vi "Grab (177x Smart Camera).vi"() -> ()   [LabVIEW 2011]
doc: "The Grab (177x Smart Camera) VI performs a high-level grab acquisition and exposes control of the sensor interface for NI 177x Series devices. A grab is appropriate for high-speed applications that process only one image at a time.\n\nUse the Sensor Parameters cluster to control attributes related to the sensor. Use the Exposure Time control (in microseconds) to precisely control the amount of time that the image sensor is sensitive to light. Use the Gain control to determine the gain of the camera. Use the Reverse X and Reverse Y to flip the image horizontally or vertically.\n\nUse the Lighting Parameters cluster to control the internal lighting controller. The internal lighting controller is precisely synchronized with the exposure of the image sensor. This guarantees that the light is on for the duration of the image exposure period.\n\nUse the Trigger Parameters cluster to configure the trigger mode of the acquisition. These settings must be configured before running the VI because they are ignored while the acquisition is active."
uses:
  <vilib>/vision/driver/IMAQdx.llb/IMAQdx Buffer Number Mode.ctl
  <vilib>/vision/driver/NI_Vision_Acquisition_Software.lvlib
  <vilib>/vision/driver/IMAQdx.llb/IMAQdx Acquisition Mode.ctl
  resource/objmgr/imaqdx.rc
panel:
  in  "SW Trigger":bool
  in  "Trigger Parameters":T1={"Trigger Mode"="Off", "Trigger Source"="External Trigger", "Fixed Frame Rate"=0.25, "Timeout (ms)"=5000, "Trigger Delay (us)"=0.0} {"Trigger Delay (us)" min=0.0 max=4295000.0; "Fixed Frame Rate" min=0.25 max=15.0}
  in  "Lighting Parameters":cluster{"Mode":string, "Current Level (mA)":dbl}={"Mode"="Off", "Current Level (mA)"=0.0} {"Current Level (mA)" min=0.0 max=0.0 step=1.0 scale=0.0..100.0}
  in  "Color Parameters":T2 {"Gamma" scale=0.0..1.0; "Blue Gain" scale=0.0..3.99; "Green Gain" scale=0.0..3.99; "Red Gain" scale=0.0..3.99}
  in  "Sensor Parameters":T3={"Exposure Time (ms)"=50.0, "Gain"=0.0, "Reverse X"=FALSE, "Reverse Y"=FALSE} {"Gain" min=0.0 max=255.0; "Exposure Time (ms)" min=0.057798999999999996 max=2101.471043 scale=0.057798999999999996..1000.0 scale format="%#_1f"}
  in  "Camera Name":refnum<k21> caption="IMAQdx Session"
  out "Image":T4(plugin-control)
  out "Frame Rate":dbl(knob) scale=0.0..100.0
  in  "Stop":bool
  # "Overview: Demonstrates how to perform a high-level grab acquisition and control of the sensor interface for NI 177x Series devices.  \nRequirements: Vision Acquisition Software, NI 177x series smart camera. For 17xx cameras, use the examples in the NI-IMAQ folder instead.\nInstructions: \n1. Open a New LabVIEW Project. Select to Add this VI to the project when prompted.\n2. Right click on the Project in the tree and select New>>Targets and Devices...\n3. Select the Smart Camera you want to run this example with, and click OK.\n4. Drag this VI from My Computer to the Smart Camera.\n5. Double click on the example under the Smart Camera, select the Camera Name, and run the VI."
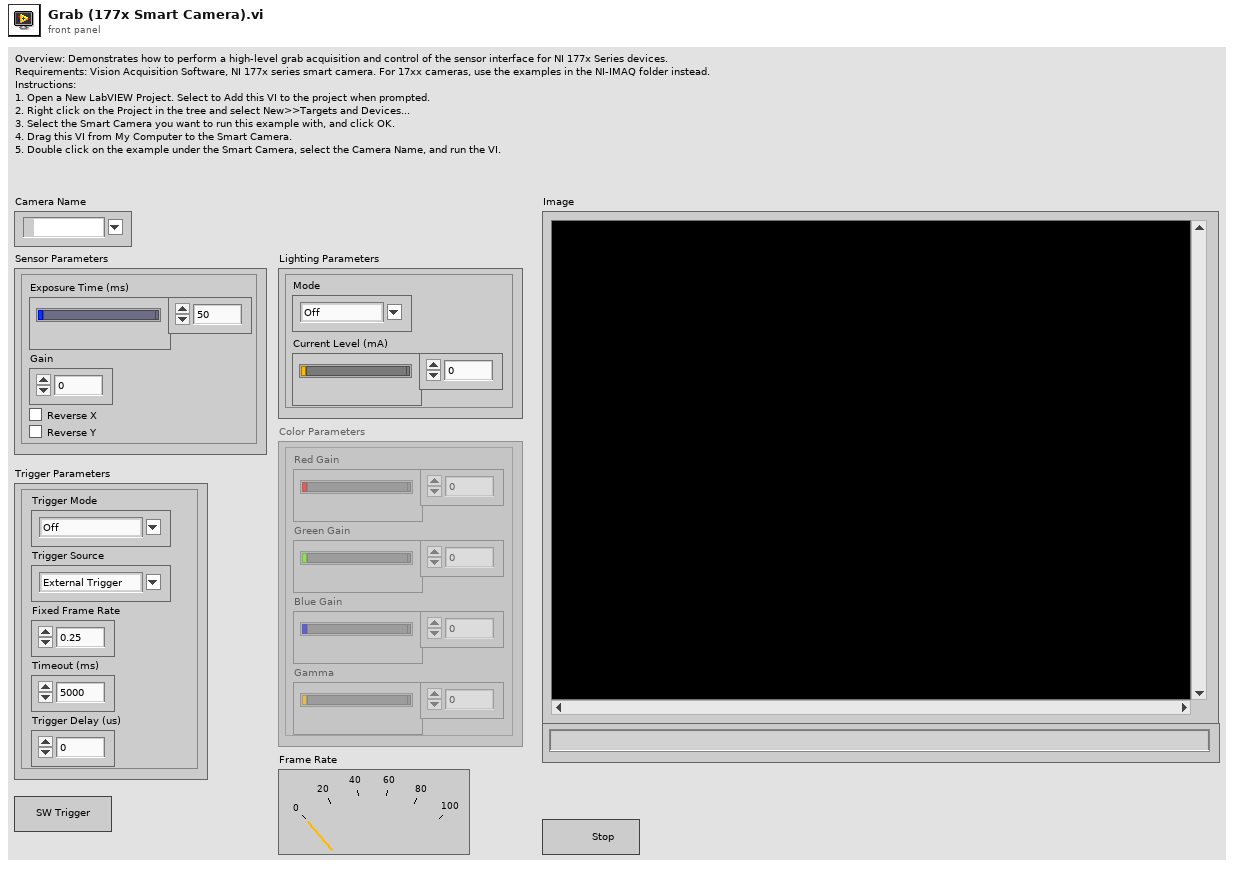
[diagram p1: front panel]
types:
  T1 = cluster{"Trigger Mode":string, "Trigger Source":string, "Fixed Frame Rate":dbl, "Timeout (ms)":u32, "Trigger Delay (us)":dbl}
  T2 = cluster{"Red Gain":dbl, "Green Gain":dbl, "Blue Gain":dbl, "Gamma":dbl}
  T3 = cluster{"Exposure Time (ms)":dbl, "Gain":dbl, "Reverse X":bool, "Reverse Y":bool}
  T4 = typedef "IMAQ Image.ctl" = refnum<image>
  T5 = enum8{"Enabled", "Disabled", "Disabled and Grayed Out"}
  T6 = typedef "NI_Vision_Acquisition_Software.lvlib/IMAQdx Acquisition Mode.ctl" = enum32{"One Shot", "Continuous"}
  T7 = typedef "IMAQdx.ctl" = refnum<k21>
  T8 = typedef "NI_Vision_Acquisition_Software.lvlib/IMAQdx Buffer Number Mode.ctl" = enum32{"Next", "Last", "Buffer Number", "Every", "Last New"}
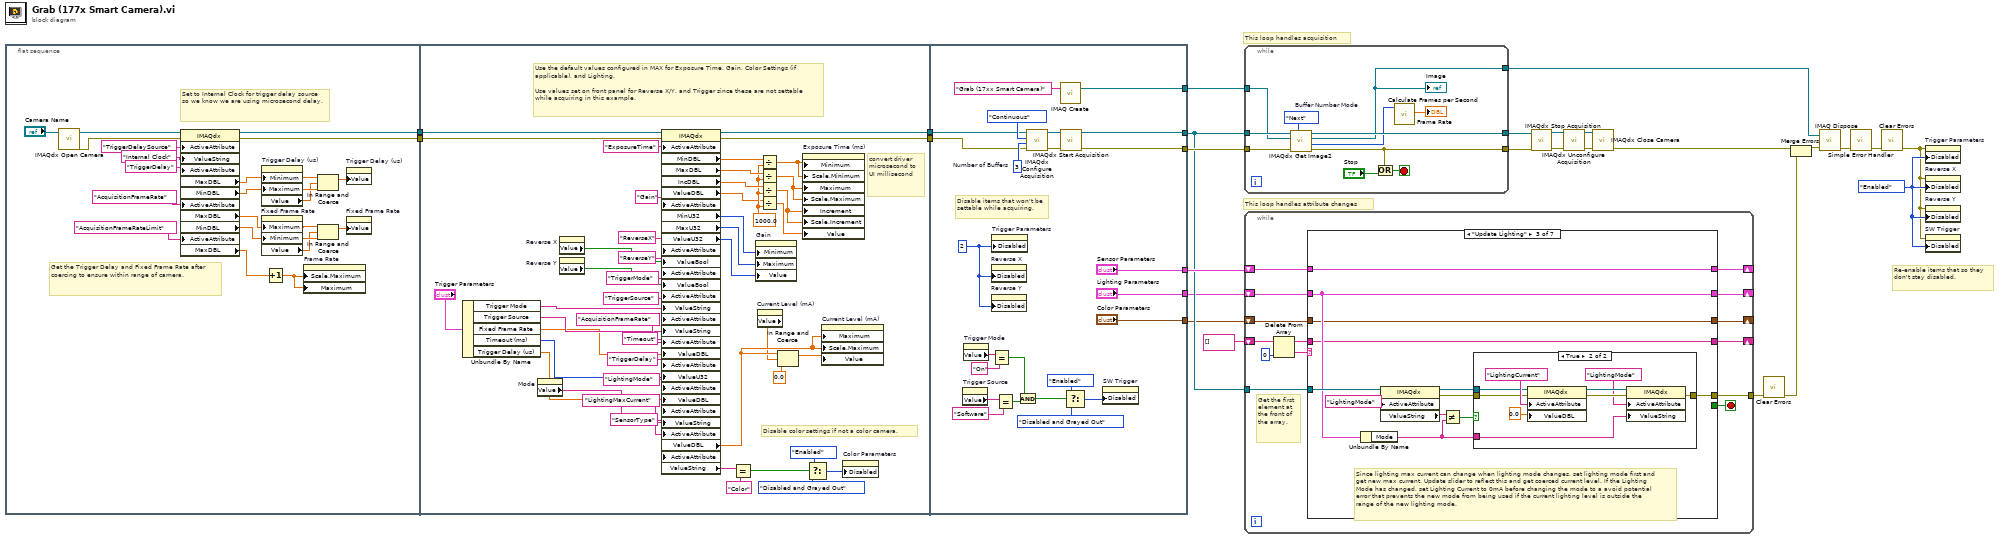
[diagram p0: block diagram]
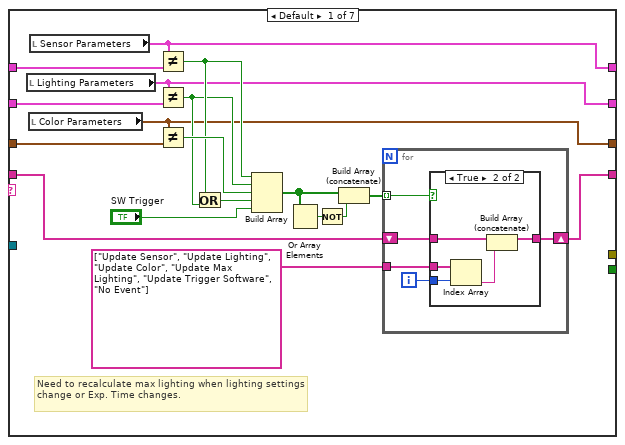
[diagram p2: hidden frame]
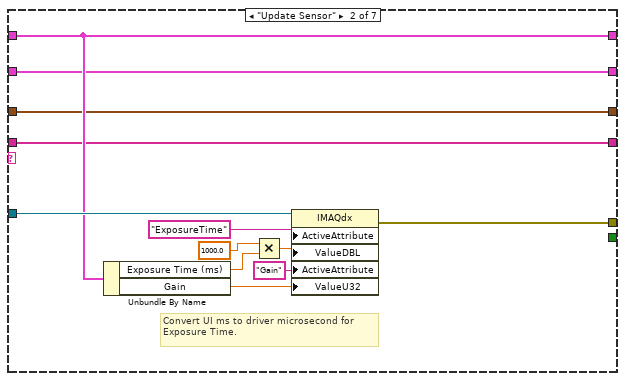
[diagram p4: hidden frame]
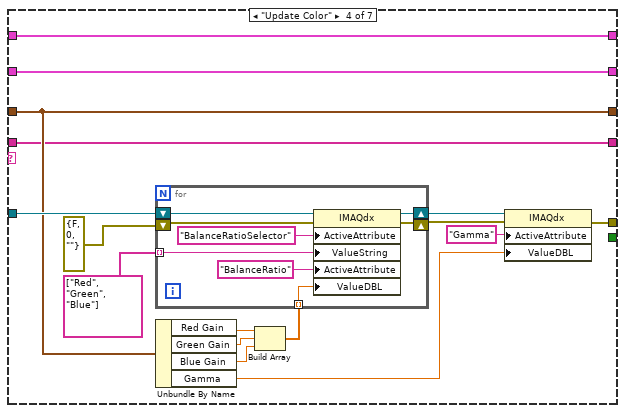
[diagram p6: hidden frame]
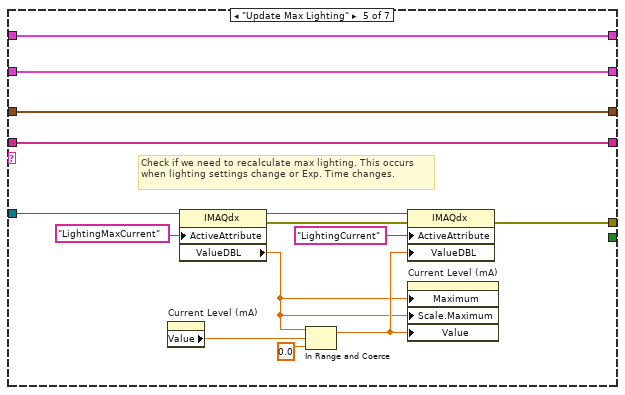
[diagram p7: hidden frame]
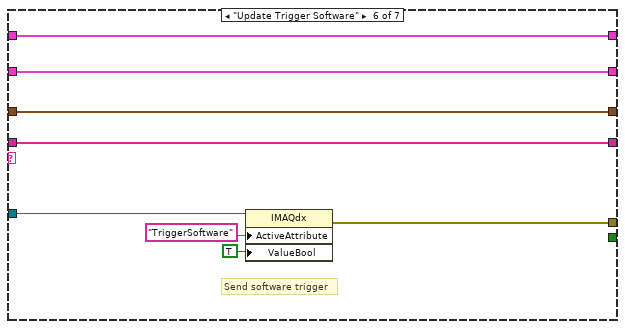
[diagram p8: hidden frame]
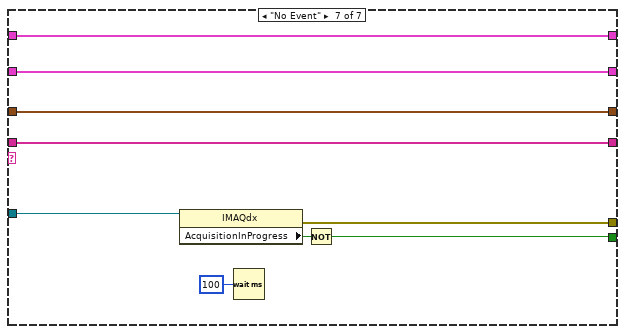
[diagram p9: hidden frame]
diagram:
  w12 = T5."Enabled" ("Disabled")
  # "Re-enable items that so they don't stay disabled."
  # "This loop handles acquisition"
  # "This loop handles attribute changes"
  n1 = flat-sequence {
    tunnel: [w30] -> w21
    tunnel: [w35] -> w20
    tunnel: w21 -> [w56]
    tunnel: [w55] -> w19
    tunnel: w20 -> [w83]
    tunnel: [w69] -> w18
    tunnel: w19 -> [w113]
    tunnel: [w111] -> w24
    tunnel: [w110] -> w26
    tunnel: ["Sensor Parameters"] -> w25
    tunnel: ["Lighting Parameters"] -> w23
    tunnel: ["Color Parameters"] -> w22
    tunnel: w18 -> [w112]
    tunnel: [w94] -> w17
    frame #0 {
      # "Get the Trigger Delay and Fixed Frame Rate after coercing to ensure within range of camera."
      # "Set to Internal Clock for trigger delay source so we know we are using microsecond delay."
      n2 = call <vilib>:"IMAQdx Open Camera.vi"("Session In"="Camera Name") -> ("error out"=w27:errorcluster, "Session Out"=w28:T7)  [unwired: 2 in, 7 out]
      n3 = property class="IMAQdx"(reference=w28, error in=w27, "ActiveAttribute"="TriggerDelaySource", "ValueString"="Internal Clock", "ActiveAttribute"="TriggerDelay", "ActiveAttribute"="AcquisitionFrameRate", "ActiveAttribute"="AcquisitionFrameRateLimit") -> (reference out=w30:T7, error out=w35:errorcluster, "MaxDBL"=w43:dbl, "MinDBL"=w42:dbl, "MaxDBL"=w38:dbl, "MinDBL"=w37:dbl, "MaxDBL"=w31:dbl)
      n4 = property on="Trigger Delay (us)" class="DigNum (strict)"("Minimum"=w43, "Maximum"=w42) -> ("Value"=w41:dbl)  [unwired: 2 in, 2 out]
      n5 = property on="Fixed Frame Rate" class="DigNum (strict)"("Maximum"=w38, "Minimum"=w37) -> ("Value"=w36:dbl)  [unwired: 2 in, 2 out]
      n6 = Increment(x=w31) -> (x+1=w32:dbl)
      n7 = property on="Frame Rate" class="Knob (strict)"("Scale.Maximum"=w32, "Maximum"=w32) -> ()  [unwired: 2 in, 2 out]
      n8 = In Range and Coerce(upper limit=w43, x=w41, lower limit=w42) -> (coerced(x)=w40:dbl)  [unwired: 1 out]
      n9 = In Range and Coerce(upper limit=w38, x=w36, lower limit=w37) -> (coerced(x)=w34:dbl)  [unwired: 1 out]
      n10 = property on="Trigger Delay (us)" class="DigNum (strict)"("Value"=w40) -> ()  [unwired: 2 in, 2 out]
      n11 = property on="Fixed Frame Rate" class="DigNum (strict)"("Value"=w34) -> ()  [unwired: 2 in, 2 out]
    }
    frame #1 {
      w63 = 1000.0 ("y")
      # "convert driver microsecond to UI millisecond"
      # "Disable color settings if not a color camera."
      # "Use the default values configured in MAX for Exposure Time, Gain, Color Settings (if applicable), and Lighting.\n\nUse values set on front panel for Reverse X/Y, and Trigger since these are not settable while acquiring in this example."
      n12 = Unbundle By Name("Trigger Parameters") -> ("Trigger Mode"=w47:string, "Trigger Source"=w51:string, "Fixed Frame Rate"=w50:dbl, "Timeout (ms)"=w49:u32, "Trigger Delay (us)"=w48:dbl)
      n13 = property on="Mode" class="CmbBox"() -> ("Value"=w78:string)  [unwired: 2 in, 2 out]
      n14 = property on="Reverse X" class="Bool (strict)"() -> ("Value"=w87:bool)  [unwired: 2 in, 2 out]
      n15 = property on="Reverse Y" class="Bool (strict)"() -> ("Value"=w86:bool)  [unwired: 2 in, 2 out]
      n16 = property class="IMAQdx"(reference=w56, error in=w83, "ActiveAttribute"="ExposureTime", "ActiveAttribute"="Gain", "ActiveAttribute"="ReverseX", "ValueBool"=w87, "ActiveAttribute"="ReverseY", "ValueBool"=w86, "ActiveAttribute"="TriggerMode", "ValueString"=w47, "ActiveAttribute"="TriggerSource", "ValueString"=w51, "ActiveAttribute"="AcquisitionFrameRate", "ValueDBL"=w50, "ActiveAttribute"="Timeout", "ValueU32"=w49, "ActiveAttribute"="TriggerDelay", "ValueDBL"=w48, "ActiveAttribute"="LightingMode", "ValueString"=w78, "ActiveAttribute"="LightingMaxCurrent", "ActiveAttribute"="SensorType") -> (reference out=w55:T7, error out=w69:errorcluster, "MinDBL"=w67:dbl, "MaxDBL"=w66:dbl, "IncDBL"=w65:dbl, "ValueDBL"=w53:dbl, "MinU32"=w92:u32, "MaxU32"=w91:u32, "ValueU32"=w90:u32, "ValueDBL"=w76:dbl, "ValueString"=w71:string)
      n17 = Equal?(x=w71, y="Color" ("x")) -> (x = y?=w68:bool)
      n18 = property on="Gain" class="DigNum (strict)"("Minimum"=w92, "Maximum"=w91, "Value"=w90) -> ()  [unwired: 2 in, 2 out]
      n19 = property on="Current Level (mA)" class="Slide (strict)"() -> ("Value"=w75:dbl)  [unwired: 2 in, 2 out]
      n20 = Divide(x=w67, y=w63) -> (x/y=w62:dbl)
      n21 = Divide(x=w66, y=w63) -> (x/y=w54:dbl)
      n22 = Divide(x=w65, y=w63) -> (x/y=w61:dbl)
      n23 = Divide(x=w53, y=w63) -> (x/y=w60:dbl)
      n24 = In Range and Coerce(upper limit=w76, x=w75, lower limit=0.0) -> (coerced(x)=w73:dbl)  [unwired: 1 out]
      n25 = property on="Exposure Time (ms)" class="Slide (strict)"("Minimum"=w62, "Scale.Minimum"=w62, "Maximum"=w54, "Scale.Maximum"=w54, "Increment"=w61, "Scale.Increment"=w61, "Value"=w60) -> ()  [unwired: 2 in, 2 out]
      n26 = Select(t=T5."Enabled" ("Disabled"), s=w68, f=T5."Disabled and Grayed Out" ("Disabled")) -> (s? t:f=w58:T5)
      n27 = property on="Current Level (mA)" class="Slide (strict)"("Maximum"=w76, "Scale.Maximum"=w76, "Value"=w73) -> ()  [unwired: 2 in, 2 out]
      n28 = property on="Color Parameters" class="Clust (strict)"("Disabled"=w58) -> ()  [unwired: 2 in, 2 out]
    }
    frame #2 {
      w106 = u8 2 ("Disabled")
      w117 = u32 3  # Number of Buffers
      # "Disable items that won't be settable while acquiring."
      n29 = property on="Trigger Source" class="CmbBox"() -> ("Value"=w103:string)  [unwired: 2 in, 2 out]
      n30 = property on="Trigger Mode" class="CmbBox"() -> ("Value"=w105:string)  [unwired: 2 in, 2 out]
      n31 = property on="Reverse X" class="Bool (strict)"("Disabled"=w106) -> ()  [unwired: 2 in, 2 out]
      n32 = property on="Reverse Y" class="Bool (strict)"("Disabled"=w106) -> ()  [unwired: 2 in, 2 out]
      n33 = Equal?(x=w105, y="On") -> (x = y?=w100:bool)
      n34 = property on="Trigger Parameters" class="Clust (strict)"("Disabled"=w106) -> ()  [unwired: 2 in, 2 out]
      n35 = Equal?(x=w103, y="Software") -> (x = y?=w101:bool)
      n36 = And(x=w100, y=w101) -> (x .and. y?=w99:bool)
      n37 = call <vilib>:"IMAQdx Configure Acquisition.vi"("error in"=w112, "Number of Buffers"=w117, "Continuous?"=IMAQdx_Acquisition_Mode."Continuous", "Session In"=w113) -> ("error out"=w115:errorcluster, "Session Out"=w114:T7)  [unwired: 6 out]
      n38 = call "IMAQ Create"("Image Name"="Grab (17xx Smart Camera)") -> ("New Image"=w94:T4)  [unwired: 3 in, 2 out]
      n39 = call <vilib>:"IMAQdx Start Acquisition.vi"("error in"=w115, "Session In"=w114) -> ("error out"=w110:errorcluster, "Session Out"=w111:T7)  [unwired: 8 out]
      n40 = Select(t=T5."Enabled" ("Disabled"), s=w99, f=T5."Disabled and Grayed Out" ("Disabled")) -> (s? t:f=w98:T5)
      n41 = property on="SW Trigger" class="Bool"("Disabled"=w98) -> ()  [unwired: 2 in, 2 out]
    }
  }
  n42 = while {
    tunnel: [w125] -> w16
    tunnel: w26 -> [w126]
    tunnel: w24 -> [w127]
    tunnel: [w121] -> w15
    tunnel: w17 -> [w120]
    tunnel: [w118] -> w14
    stop <- w128 stop-if-true
    w124 = IMAQdx_Buffer_Number_Mode."Next"  # Buffer Number Mode
    n43 = call <vilib>:"IMAQdx Get Image2.vi"("Buffer Number Mode (Next)"=w124, "error in"=w126, "Image In"=w120, "Session In"=w127) -> ("error out"=w121:errorcluster, "Buffer Number Out"=w119:u32, "Image Out"=w118:T4, "Session Out"=w125:T7)  [unwired: 4 in]
    "Image" <- w118
    n44 = Or(x=w121, y="Stop") -> (x .or. y?=w128:bool)
    n45 = call <vilib>:"Calculate Frames per Second.vi"("Buffer Number"=w119) -> ("Processed Frames/s"=→"Frame Rate":dbl)  [unwired: 8 in, 2 out]
  }
  n46 = while {
    shift-right: [w141] -> _
    shift-left: w25 -> [w142]
    shift-right: [w139] -> _
    shift-left: w23 -> [w132]
    shift-right: [w138] -> _
    shift-left: w22 -> [w131]
    tunnel: w24 -> [w140]
    shift-right: [w130] -> _
    shift-left: string[] [] -> [w135]
    tunnel: [w129] -> w7
    stop <- w137 stop-if-true
    # "Get the first element at the front of the array."
    n47 = Delete From Array(array=w135, index=0) -> (deleted portion=w134:string, array with subset deleted=w133:string[])  [unwired: 1 in]
    n48 = case shown="\"Update Lighting\"" w134 {
      tunnel: w142 -> [w160 w176 w192 w211 w234 w248 w254]
      tunnel: [w149 w176 w192 w211 w234 w248 w254] -> w141
      tunnel: w140 -> [_ w183 w195 w221 w243 w251 w259]
      tunnel: [w148 w175 w193 w210 w233 w247 w255] -> w139
      tunnel: [w147 w174 w191 w220 w232 w246 w256] -> w138
      tunnel: [_ _ _ _ _ _ w252] -> w137
      tunnel: w131 -> [w158 w174 w191 w220 w232 w246 w256]
      tunnel: w133 -> [w153 w173 w190 w209 w231 w245 w257]
      tunnel: w132 -> [w159 w175 w193 w210 w233 w247 w255]
      tunnel: [w145 w173 w190 w209 w231 w245 w257] -> w130
      tunnel: [_ w172 w184 w207 w230 w244 w253] -> w129
      frame Default {
        # "Need to recalculate max lighting when lighting settings change or Exp. Time changes."
        n49 = local read "Lighting Parameters"() -> (w148:cluster{"Mode":string, "Current Level (mA)":dbl})
        n50 = local read "Color Parameters"() -> (w147:T2)
        n51 = local read "Sensor Parameters"() -> (w149:T3)
        n52 = Not Equal?(x=w149, y=w160) -> (x != y?=w152:bool)
        n53 = Not Equal?(x=w148, y=w159) -> (x != y?=w151:bool)
        n54 = Not Equal?(x=w147, y=w158) -> (x != y?=w157:bool)
        n55 = Or(x=w152, y=w151) -> (x .or. y?=w156:bool)
        n56 = Build Array(w152, w151, w157, w156, "SW Trigger") -> (w155:bool[])
        n57 = Or Array Elements(Boolean array=w155) -> (logical OR=w144:bool)
        n58 = Not(x=w144) -> (.not. x?=w143:bool)
        n59 = Build Array (concatenate)(w155, w143) -> (w154:bool[])
        n60 = for {
          tunnel: w154 -> [w165] mode=indexing
          shift-right: [w163] -> w145
          shift-left: w153 -> [w164]
          tunnel: string[] ["Update Sensor", "Update Lighting", "Update Color", "Update Max Lighting", "Update Trigger Software", "No Event"] -> [w162]
          i -> [w161]
          n61 = case shown="True" w165 {
            tunnel: w164 -> [w166 w171]
            tunnel: w161 -> [_ w170]
            tunnel: [w166 w168] -> w163
            tunnel: w162 -> [_ w167]
            frame False {
            }
            frame True {
              n62 = Index Array(array=w167, index=w170) -> (element=w169:string)
              n63 = Build Array (concatenate)(w171, w169) -> (w168:string[])
            }
          }
        }
      }
      frame "Update Sensor" {
        # "Convert UI ms to driver microsecond for Exposure Time."
        n64 = Unbundle By Name(w176) -> ("Exposure Time (ms)"=w178:dbl, "Gain"=w182:dbl)
        n65 = Multiply(x=1000.0, y=w178) -> (x*y=w179:dbl)
        n66 = property class="IMAQdx"(reference=w183, "ActiveAttribute"="ExposureTime", "ValueDBL"=w179, "ActiveAttribute"="Gain", "ValueU32"=w182) -> (error out=w172:errorcluster)  [unwired: 1 in, 1 out]
      }
      frame "Update Lighting" {
        # "Since lighting max current can change when lighting mode changes, set lighting mode first and get new max current. Update slider to reflect this and get coerced current level. If the Lighting Mode has changed, set Lighting Current to 0mA before changing the mode to a avoid potential error that prevents the new mode from being used if the current lighting level is outside the range of the new lighting mode."
        n67 = Unbundle By Name(w193) -> ("Mode"=w187:string)
        n68 = property class="IMAQdx"(reference=w195, "ActiveAttribute"="LightingMode") -> (reference out=w186:T7, error out=w185:errorcluster, "ValueString"=w189:string)  [unwired: 1 in]
        n69 = Not Equal?(x=w189, y=w187) -> (x != y?=w188:bool)
        n70 = case shown="True" w188 {
          tunnel: w186 -> [_ w204]
          tunnel: w185 -> [w196 w203]
          tunnel: [w196 w199] -> w184
          tunnel: w187 -> [_ w197]
          frame False {
          }
          frame True {
            n71 = property class="IMAQdx"(reference=w204, error in=w203, "ActiveAttribute"="LightingCurrent", "ValueDBL"=0.0) -> (reference out=w201:T7, error out=w200:errorcluster)
            n72 = property class="IMAQdx"(reference=w201, error in=w200, "ActiveAttribute"="LightingMode", "ValueString"=w197) -> (error out=w199:errorcluster)  [unwired: 1 out]
          }
        }
      }
      frame "Update Color" {
        n73 = Unbundle By Name(w220) -> ("Red Gain"=w218:dbl, "Green Gain"=w217:dbl, "Blue Gain"=w216:dbl, "Gamma"=w208:dbl)
        n74 = Build Array(w218, w217, w216) -> (w215:dbl[])
        n75 = for {
          tunnel: string[] ["Red", "Green", "Blue"] -> [w226] mode=indexing
          tunnel: w215 -> [w225] mode=indexing
          shift-right: [w224] -> w214
          shift-left: w221 -> [w229]
          shift-right: [w222] -> w212
          shift-left: errorcluster {"status"=FALSE, "code"=0, "source"=""} ("error out") -> [w223]
          n76 = property class="IMAQdx"(reference=w229, error in=w223, "ActiveAttribute"="BalanceRatioSelector", "ValueString"=w226, "ActiveAttribute"="BalanceRatio", "ValueDBL"=w225) -> (reference out=w224:T7, error out=w222:errorcluster)
        }
        n77 = property class="IMAQdx"(reference=w214, error in=w212, "ActiveAttribute"="Gamma", "ValueDBL"=w208) -> (error out=w207:errorcluster)  [unwired: 1 out]
      }
      frame "Update Max Lighting" {
        # "Check if we need to recalculate max lighting. This occurs when lighting settings change or Exp. Time changes."
        n78 = property on="Current Level (mA)" class="Slide (strict)"() -> ("Value"=w236:dbl)  [unwired: 2 in, 2 out]
        n79 = property class="IMAQdx"(reference=w243, "ActiveAttribute"="LightingMaxCurrent") -> (reference out=w239:T7, error out=w235:errorcluster, "ValueDBL"=w237:dbl)  [unwired: 1 in]
        n80 = In Range and Coerce(upper limit=w237, x=w236, lower limit=0.0) -> (coerced(x)=w240:dbl)  [unwired: 1 out]
        n81 = property class="IMAQdx"(reference=w239, error in=w235, "ActiveAttribute"="LightingCurrent", "ValueDBL"=w240) -> (error out=w230:errorcluster)  [unwired: 1 out]
        n82 = property on="Current Level (mA)" class="Slide (strict)"("Maximum"=w237, "Scale.Maximum"=w237, "Value"=w240) -> ()  [unwired: 2 in, 2 out]
      }
      frame "Update Trigger Software" {
        # "Send software trigger"
        n83 = property class="IMAQdx"(reference=w251, "ActiveAttribute"="TriggerSoftware", "ValueBool"=TRUE) -> (error out=w244:errorcluster)  [unwired: 1 in, 1 out]
      }
      frame "No Event" {
        n84 = property class="IMAQdx"(reference=w259) -> (error out=w253:errorcluster, "AcquisitionInProgress"=w258:bool)  [unwired: 1 in, 1 out]
        n85 = Wait (ms)(milliseconds to wait=u32 100) -> ()  [unwired: 1 out]
        n86 = Not(x=w258) -> (.not. x?=w252:bool)
      }
    }
  }
  n87 = call <vilib>:"IMAQdx Stop Acquisition.vi"("error in"=w15, "Session In"=w16) -> ("error out"=w11:errorcluster, "Session Out"=w10:T7)  [unwired: 8 out]
  n88 = call <vilib>:"IMAQdx Unconfigure Acquisition.vi"("error in"=w11, "Session In"=w10) -> ("error out"=w8:errorcluster, "Session Out"=w9:T7)  [unwired: 8 out]
  n89 = call <vilib>:"IMAQdx Close Camera.vi"("error in"=w8, "Session In"=w9) -> ("error out"=w6:errorcluster)  [unwired: 9 out]
  n90 = call <vilib>:"Clear Errors.vi"("error in (no error)"=w7) -> ("error out"=w5:errorcluster)  [unwired: 6 in]
  n91 = Merge Errors(w6, w5) -> (w4:errorcluster)
  n92 = call "IMAQ Dispose"("Image"=w14, "error in (no error)"=w4) -> ("error out"=w2:errorcluster)  [unwired: 4 in]
  n93 = call <vilib>:"Simple Error Handler.vi"("error in (no error)"=w2) -> ("error out"=w1:errorcluster)  [unwired: 4 in, 4 out]
  n94 = call <vilib>:"Clear Errors.vi"("error in (no error)"=w1) -> ("error out"=w3:errorcluster)  [unwired: 6 in]
  n95 = property on="Trigger Parameters" class="Clust (strict)"(error in=w3, "Disabled"=w12) -> ()  [unwired: 1 in, 2 out]
  n96 = property on="Reverse X" class="Bool (strict)"(error in=w3, "Disabled"=w12) -> ()  [unwired: 1 in, 2 out]
  n97 = property on="Reverse Y" class="Bool (strict)"(error in=w3, "Disabled"=w12) -> ()  [unwired: 1 in, 2 out]
  n98 = property on="SW Trigger" class="Bool"(error in=w3, "Disabled"=w12) -> ()  [unwired: 1 in, 2 out]
